vi "_PC_Pub_ExpCondi_SubVI_Get_LaserParameter.vi"(8 "error in (no error)":errorcluster, 11 "result string":string) -> (0 "error out":errorcluster, 3 "output cluster":T1)   [LabVIEW 2018]
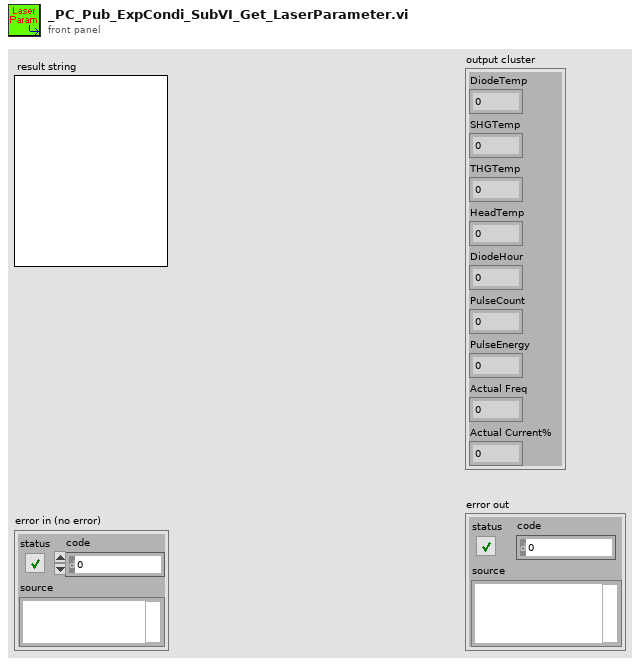
[diagram p1: front panel]
types:
  T1 = cluster{"DiodeTemp":dbl, "SHGTemp":dbl, "THGTemp":dbl, "HeadTemp":dbl, "DiodeHour":dbl, "PulseCount":dbl, "PulseEnergy":dbl, "Actual Freq":dbl, "Actual Current%":dbl}
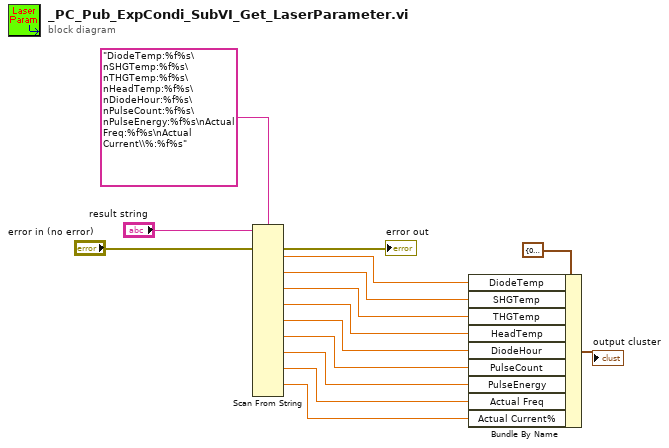
[diagram p0: block diagram]
diagram:
  n1 = Scan From String(format string="DiodeTemp:%f%s\nSHGTemp:%f%s\nTHGTemp:%f%s\nHeadTemp:%f%s\nDiodeHour:%f%s\nPulseCount:%f%s\nPulseEnergy:%f%s\nActual Freq:%f%s\nActual Current\\%:%f%s", input string="result string", error in="error in (no error)") -> (error out=→"error out":errorcluster, output 1=w9:dbl, output 3=w8:dbl, output 5=w7:dbl, output 7=w6:dbl, output 9=w5:dbl, output 11=w4:dbl, output 13=w3:dbl, output 15=w2:dbl, output 17=w1:dbl)  [unwired: 28 in, 2 out]
  n2 = Bundle By Name(cluster=T1 {"DiodeTemp"=0.0, "SHGTemp"=0.0, "THGTemp"=0.0, "HeadTemp"=0.0, "DiodeHour"=0.0, "PulseCount"=0.0, "PulseEnergy"=0.0, "Actual Freq"=0.0, "Actual Current%"=0.0}, "DiodeTemp"=w9, "SHGTemp"=w8, "THGTemp"=w7, "HeadTemp"=w6, "DiodeHour"=w5, "PulseCount"=w4, "PulseEnergy"=w3, "Actual Freq"=w2, "Actual Current%"=w1) -> (→"output cluster":T1)
